vi "ma_Updatet0.vi"   [LabVIEW 2020, in "NI_MABase.lvlib"]
uses:
  NI_MABase.lvlib
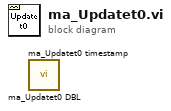
[diagram p0: block diagram]
diagram:
  n1 = call "ma_Updatet0 DBL.vi"() -> ()  [unwired: 4 in, 2 out]
  n2 = call "ma_Updatet0 timestamp.vi"() -> ()  [unwired: 4 in, 2 out]
